vi "Get Bias Voltage.vi"(8 "error in (no error)":errorcluster, 9 "Channel":u32, 11 "Instrument.VSource in":refnum<class "Instrument.VSource.lvclass">) -> (0 "error out":errorcluster, 2 "Bias Voltage (V)":dbl, 3 "Instrument.VSource out":refnum<class "Instrument.VSource.lvclass">)   [LabVIEW 2019, in "Instrument.VSource.lvclass"]
uses:
  Instrument.VSource.lvclass
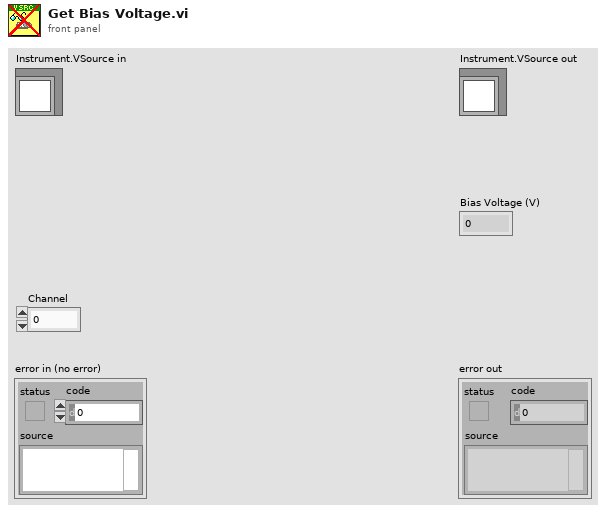
[diagram p1: front panel]
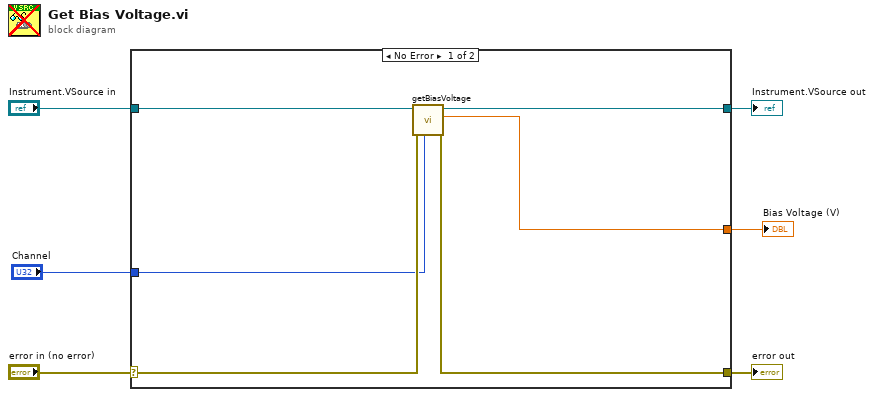
[diagram p0: block diagram]
diagram:
  n1 = case shown="No Error" "error in (no error)" {
    selector: "error in (no error)" -> [w12 w14]
    tunnel: [w11 w14] -> w5
    tunnel: [w9 w13] -> w3
    tunnel: "Instrument.VSource in" -> [w8 w13]
    tunnel: "Channel" -> [w7 _]
    tunnel: [w10 _] -> w1
    frame No Error {
      n2 = call-dynamic "getBiasVoltage.vi"("Channel"=w7, "error in (no error)"=w12, "Instrument.VSource in"=w8) -> ("error out"=w11:errorcluster, "Bias Voltage (V)"=w10:dbl, "Instrument.VSource out"=w9:refnum<class "Instrument.VSource.lvclass">)  [unwired: 6 in]
    }
    frame Error {
    }
  }
  "error out" <- w5
  "Instrument.VSource out" <- w3
  "Bias Voltage (V)" <- w1
